vi "GetWebcamsAsync.vi"   [LabVIEW 2015]
uses:
  Anemometry/Anemometry Sub Vis/Globals/Constants_global.vi
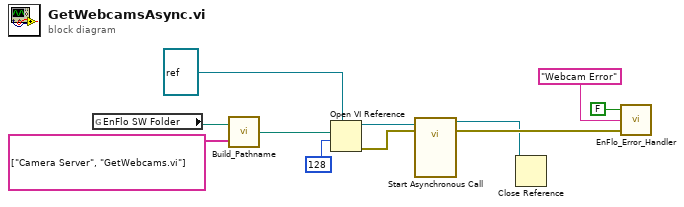
[diagram p0: block diagram]
diagram:
  n1 = global read "Constants_global.vi" "EnFlo SW Folder"() -> (w3:path)
  n2 = call "Build_Pathname.vi"("PathElements"=string[] ["Camera Server", "GetWebcams.vi"] ("array of strings"), "PathnameIn"=w3) -> ("AppendedPath"=w11:path)
  n3 = Open VI Reference(type specifier VI Refnum (for type only)=refnum<vi> refnum, vi path=w11, options=128) -> (vi reference=w4:refnum<vi>, error out=w7:errorcluster)  [unwired: 3 in]
  n4 = call-by-ref "Start Asynchronous Call"(reference=w4, error in=w7) -> (reference out=w1:refnum<vi>, error out=w8:errorcluster)  [unwired: 11 in]
  n5 = Close Reference(reference=w1) -> ()  [unwired: 1 in, 1 out]
  n6 = call "EnFlo_Error_Handler.vi"("error in (no error)"=w8, "Error Type"="Webcam Error", "Dialog Box (T)"=FALSE) -> ()  [unwired: 3 out]
